vi "Set Property by Name.vi"(8 "error in (no error)":errorcluster, 9 "Value":variant, 10 "Name":string, 11 "Tag in":refnum<class "Tag.lvclass">) -> (0 "error out":errorcluster, 2 "Replaced?":bool, 3 "Tag out":refnum<class "Tag.lvclass">)   [LabVIEW 2018, in "Tag Engine.lvlib" / "Tag.lvclass"]
doc: "_SubVI_"
uses:
  Tag.lvclass
  Tag.lvclass/Tag.ctl
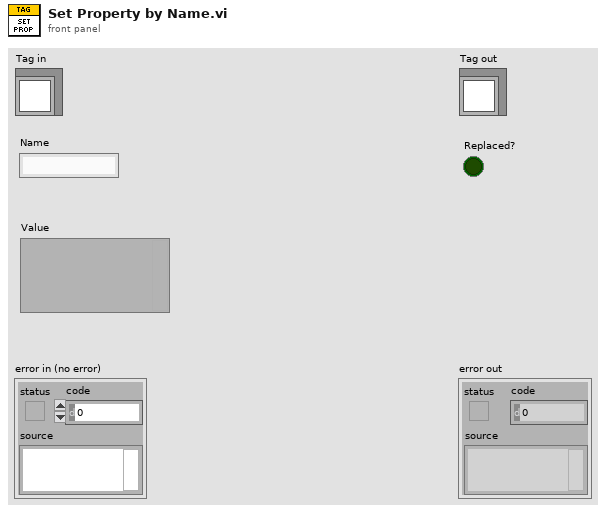
[diagram p1: front panel]
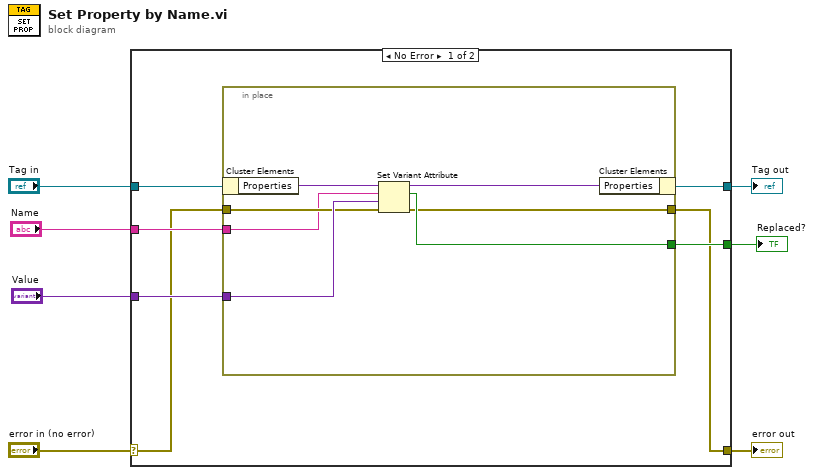
[diagram p0: block diagram]
diagram:
  n1 = case shown="No Error" "error in (no error)" {
    selector: "error in (no error)" -> [w9 w23]
    tunnel: [w8 w23] -> w6
    tunnel: [w13 w22] -> w4
    tunnel: "Tag in" -> [w14 w22]
    tunnel: "Name" -> [w12 _]
    tunnel: "Value" -> [w11 _]
    tunnel: [w10 _] -> w1
    frame No Error {
      n2 = in-place {
        in-place-border: w12 -> [w15]
        in-place-border: w11 -> [w21]
        in-place-border: [w18] -> w10
        in-place-border: w9 -> [w17]
        in-place-border: [w16] -> w8
        n3 = in-place-cluster #1(w14) -> ("Properties"=w20:variant)
        n4 = Set Variant Attribute(Variant=w20, name=w15, value=w21, error in=w17) -> (Variant out=w19:variant, replaced=w18:bool, error out=w16:errorcluster)
        n5 = in-place-cluster #1("Properties"=w19) -> (w13:refnum<class "Tag.lvclass">)
      }
    }
    frame Error {
    }
  }
  "error out" <- w6
  "Tag out" <- w4
  "Replaced?" <- w1
